vi "Get Crafting Stations.vi"(8 "error in (no error)":errorcluster, 11 "Item in":refnum<class "Item.lvclass">) -> (0 "error out":errorcluster, 2 "Stations":T1[](array[typedef]), 3 "Item out":refnum<class "Item.lvclass">)   [LabVIEW 2020, in "Item.lvclass"]
uses:
  Item.lvclass
  Craft Station.ctl
  Workstation/Workstation.lvclass
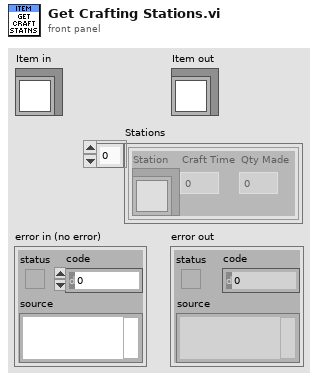
[diagram p1: front panel]
types:
  T1 = typedef "Item.lvclass/Craft Station.ctl" = cluster{"Station":refnum<class "Workstation.lvclass">, "Craft Time":dbl, "Qty Made":dbl}
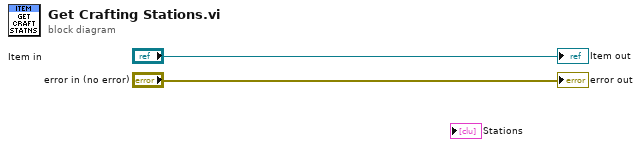
[diagram p0: block diagram]
diagram:
  "error out" <- "error in (no error)"
  "Item out" <- "Item in"
